vi "Status Pump Status.vi"(5 "Retry Attempts (0)":i32 min=0, 7 "Fast Comms (F)":bool, 8 "error in (no error)":errorcluster, 11 "VISA resource name":refnum<visa-resource-name>) -> (0 "error out":errorcluster, 2 "Status Cluster":T1, 3 "VISA resource name out":refnum<visa-resource-name>)   [LabVIEW 2020, in "ChromTech Series I Drivers.lvlib"]
doc: "Returns the current pump information. Series I will always return no pressure faults."
uses:
  <instrlib>/RxnRover/ChromtechSeriesIDriver/ChromTech Series I Drivers.lvlib
panel:
  out "Response":string
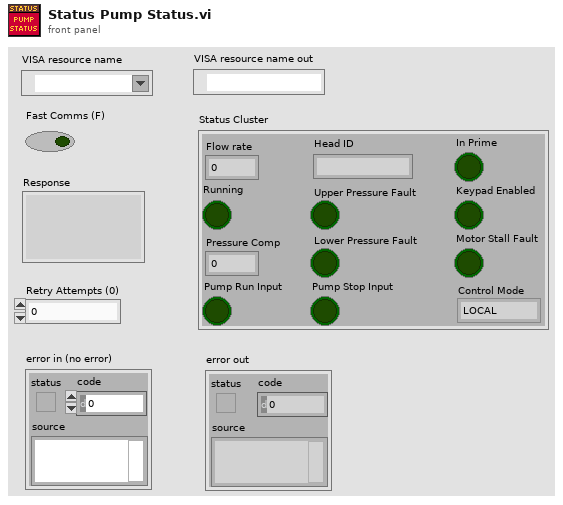
[diagram p1: front panel]
types:
  T1 = cluster{"Flow rate":dbl, "Running":bool, "Pressure Comp":i32, "Head ID":string, "Upper Pressure Fault":bool, "Lower Pressure Fault":bool, "In Prime":bool, "Keypad Enabled":bool, "Motor Stall Fault":bool, "Pump Run Input":bool, "Pump Stop Input":bool, "Control Mode":enum16{"LOCAL", "REMOTE"}}
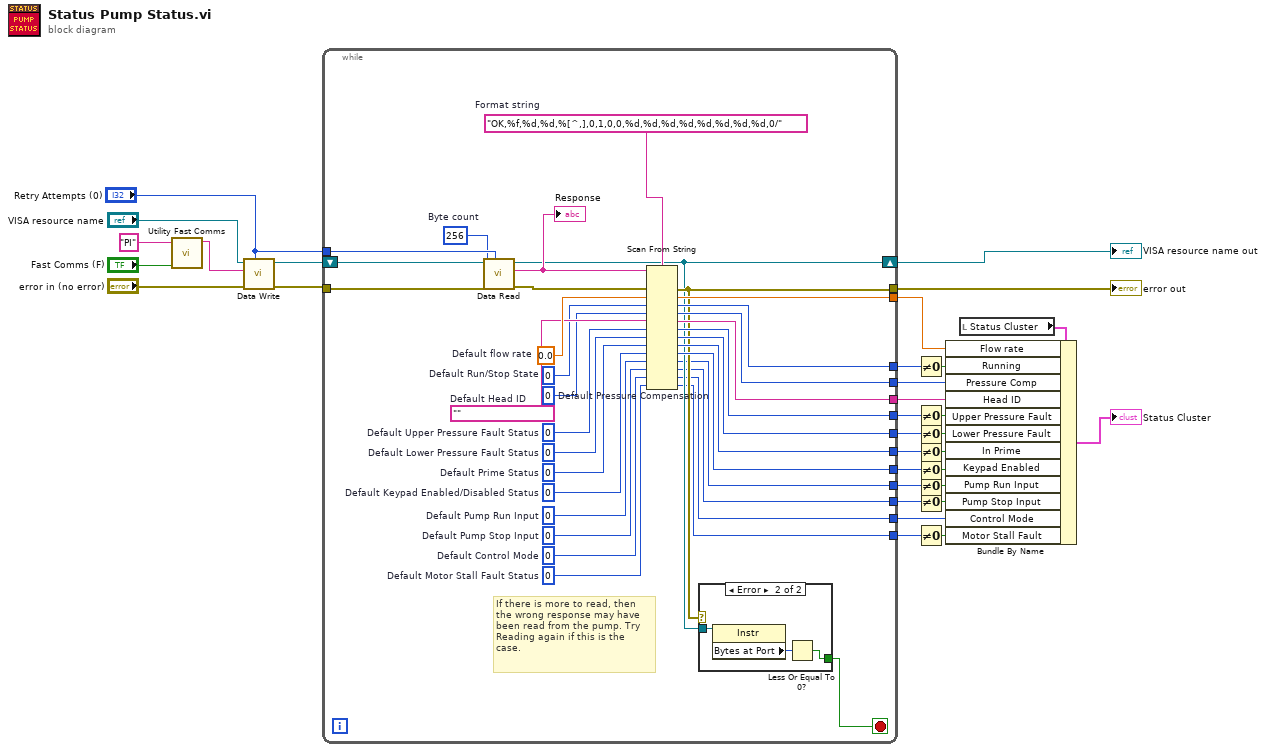
[diagram p0: block diagram]
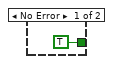
[diagram p2: hidden frame]
diagram:
  n1 = call <instrlib>:"Utility Fast Comms.vi"("Fast Comms"="Fast Comms (F)", "Command"="PI" ("command")) -> ("Fast Command"=w28:string)  [unwired: 9 in]
  n2 = call <instrlib>:"Data Write.vi"("Retry Attempts (0)"="Retry Attempts (0)", "error in (no error)"="error in (no error)", "Command"=w28, "VISA Refnum in"="VISA resource name") -> ("error out"=w10:errorcluster, "VISA Refnum out"=w9:refnum<visa-resource-name>)  [unwired: 6 in]
  n3 = while {
    tunnel: [w60] -> w25
    tunnel: [w59] -> w19
    tunnel: [w58] -> w18
    tunnel: [w57] -> w17
    tunnel: [w56] -> w16
    tunnel: [w55] -> w15
    tunnel: [w54] -> w14
    tunnel: [w53] -> w13
    tunnel: [w39] -> w12
    tunnel: "Retry Attempts (0)" -> [w47]
    shift-right: [w42] -> w7
    shift-left: w9 -> [w44]
    tunnel: w10 -> [w46]
    tunnel: [w43] -> w8
    tunnel: [w35] -> w5
    tunnel: [w34] -> w2
    tunnel: [w33] -> w1
    stop <- w41 stop-if-true
    w36 = 0  # Default Pump Run Input
    w37 = 0  # Default Pump Stop Input
    w38 = 0  # Default Control Mode
    w45 = u32 256  # Byte count
    w40 = 0  # Default Motor Stall Fault Status
    w50 = 0  # Default Keypad Enabled/Disabled Status
    w51 = 0  # Default Prime Status
    w52 = 0  # Default Lower Pressure Fault Status
    w61 = 0  # Default Pressure Compensation
    w62 = 0  # Default Run/Stop State
    w63 = 0  # Default Upper Pressure Fault Status
    w64 = ""  # Default Head ID
    w65 = 0.0  # Default flow rate
    w66 = "OK,%f,%d,%d,%[^,],0,1,0,0,%d,%d,%d,%d,%d,%d,%d,%d,0/"  # Format string
    # "If there is more to read, then\nthe wrong response may have\nbeen read from the pump. Try\nReading again if this is the\ncase."
    n4 = call <instrlib>:"Data Read.vi"("Retry Attempts (0)"=w47, "error in (no error)"=w46, "Bytes to read"=w45, "VISA Refnum in"=w44) -> ("error out"=w49:errorcluster, "read buffer"=w48:string, "VISA Refnum out"=w42:refnum<visa-resource-name>)  [unwired: 5 in]
    "Response" <- w48
    n5 = Scan From String(format string=w66, input string=w48, error in=w49, default 1=w65, default 2=w62, default 3=w61, default 4=w64, default 5=w63, default 6=w52, default 7=w51, default 8=w50, default 9=w36, default 10=w37, default 11=w38, default 12=w40) -> (error out=w43:errorcluster, output 1=w60:dbl, output 2=w59:i32, output 3=w58:i32, output 4=w57:string, output 5=w56:i32, output 6=w55:i32, output 7=w54:i32, output 8=w53:i32, output 9=w34:i32, output 10=w33:i32, output 11=w35:i32, output 12=w39:i32)  [unwired: 1 in, 2 out]
    n6 = case shown="Error" w43 {
      tunnel: w42 -> [_ w70]
      tunnel: [TRUE w68] -> w41
      frame No Error {
      }
      frame Error {
        n7 = property class="Instr"(reference=w70) -> ("Bytes at Port"=w69:u32)  [unwired: 1 in, 2 out]
        n8 = Less Or Equal To 0?(x=w69) -> (x <= 0?=w68:bool)
      }
    }
  }
  "VISA resource name out" <- w7
  "error out" <- w8
  n9 = Not Equal To 0?(x=w19) -> (x != 0?=w24:bool)
  n10 = Not Equal To 0?(x=w16) -> (x != 0?=w23:bool)
  n11 = Not Equal To 0?(x=w15) -> (x != 0?=w22:bool)
  n12 = Not Equal To 0?(x=w14) -> (x != 0?=w21:bool)
  n13 = Not Equal To 0?(x=w13) -> (x != 0?=w20:bool)
  n14 = Not Equal To 0?(x=w2) -> (x != 0?=w4:bool)
  n15 = Not Equal To 0?(x=w1) -> (x != 0?=w3:bool)
  n16 = Not Equal To 0?(x=w12) -> (x != 0?=w6:bool)
  n17 = local read "Status Cluster"() -> (w27:T1)
  n18 = Bundle By Name(cluster=w27, "Flow rate"=w25, "Running"=w24, "Pressure Comp"=w18, "Head ID"=w17, "Upper Pressure Fault"=w23, "Lower Pressure Fault"=w22, "In Prime"=w21, "Keypad Enabled"=w20, "Pump Run Input"=w4, "Pump Stop Input"=w3, "Control Mode"=w5, "Motor Stall Fault"=w6) -> (→"Status Cluster":T1)
